vi "CRYUpdate Unicode MultCol Listbox Data.vi"(5 "Interpret as Unicode (T)":bool=TRUE, 6 "error in (no error)":errorcluster, 8 "Data[]":string[][](array[string]), 9 "Multicolumn Listbox Ref":refnum<vi>) -> (0 "error out":errorcluster, 3 "Multicolumn Listbox Ref":refnum<vi>)   [LabVIEW 2013]
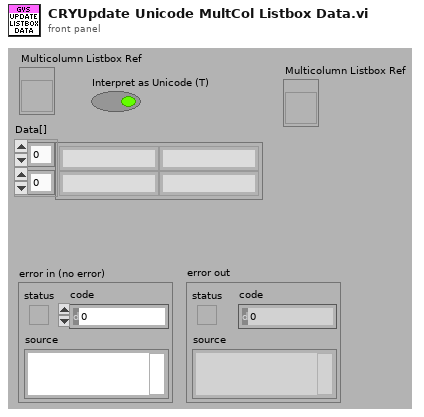
[diagram p1: front panel]
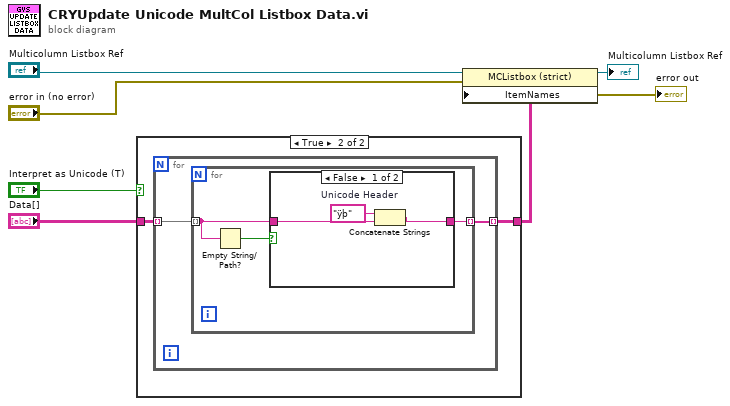
[diagram p0: block diagram]
diagram:
  n1 = case shown="True" "Interpret as Unicode (T)" {
    tunnel: "Data[]" -> [w8 w10]
    tunnel: [w8 w9] -> w1
    frame False {
    }
    frame True {
      n2 = for {
        tunnel: w10 -> [w12] mode=indexing
        tunnel: [w11] -> w9 mode=indexing
        n3 = for {
          tunnel: w12 -> [w14] mode=indexing
          tunnel: [w15] -> w11 mode=indexing
          n4 = Empty String/Path?(string/path=w14) -> (empty?=w13:bool)
          n5 = case shown="False" w13 {
            tunnel: [w18 w19] -> w15
            tunnel: w14 -> [w16 w19]
            frame False {
              w17 = "ÿþ"  # Unicode Header
              n6 = Concatenate Strings(w17, w16) -> (w18:string)
            }
            frame True {
            }
          }
        }
      }
    }
  }
  n7 = property class="MCListbox (strict)"(reference="Multicolumn Listbox Ref", error in="error in (no error)", "ItemNames"=w1) -> (reference out=→"Multicolumn Listbox Ref":refnum<vi>, error out=→"error out":errorcluster)
